vi "getDAC.vi"(3 "error in (no error)":errorcluster, 4 "DAC number":u8=2 min=1 max=8, 5 "VISA resource name IN":refnum<visa-resource-name>="COM1") -> (0 "error out":errorcluster, 1 "DAC read (mV)":dbl, 2 "VISA resource name OUT":refnum<visa-resource-name>="COM1")   [LabVIEW 2011]
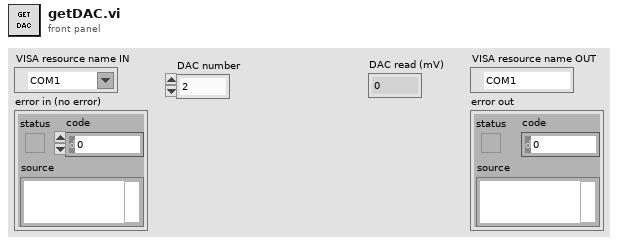
[diagram p1: front panel]
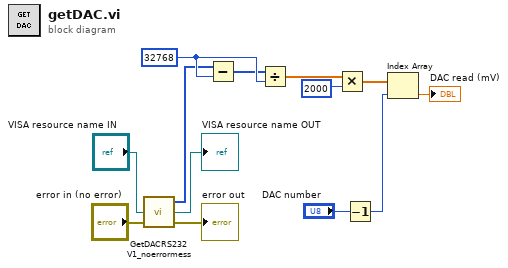
[diagram p0: block diagram]
diagram:
  w12 = 32768
  n1 = call "GetDACRS232 V1_noerrormess.vi"("error in (no error)"="error in (no error)", "VISA resource name IN"="VISA resource name IN") -> ("error out"=→"error out":errorcluster, "VISA resource name OUT"=→"VISA resource name OUT":refnum<visa-resource-name>, "DAC data out\n(hexadecimaal)"=w1:u16[])  [unwired: 1 in]
  n2 = Subtract(x=w1, y=w12) -> (x-y=w11:i32[])
  n3 = Divide(x=w11, y=w12) -> (x/y=w13:dbl[])
  n4 = Multiply(x=w13, y=2000) -> (x*y=w10:dbl[])
  n5 = Decrement(x="DAC number") -> (x-1=w8:u8)
  n6 = Index Array(array=w10, index=w8) -> (element=→"DAC read (mV)":dbl)
